vi "Rising Edge Detect (SubVI).vi"(11 "Input":bool=TRUE) -> (3 "Rising Edge?":bool)   [LabVIEW 2015]
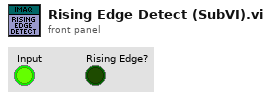
[diagram p1: front panel]
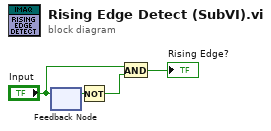
[diagram p0: block diagram]
diagram:
  n1 = feedback #1() -> (w2:bool)  [unwired: 1 in]
  n2 = feedback-in #1("Input") -> ()
  n3 = Not(x=w2) -> (.not. x?=w1:bool)
  n4 = And(x="Input", y=w1) -> (x .and. y?=→"Rising Edge?":bool)
